vi "计算合并值32位.vi"(1 "数值LL":u8, 2 "数值L":u8, 3 "数值H":u8, 4 "数值HH":u8) -> (0 "合并数值":i32)   [LabVIEW 2016]
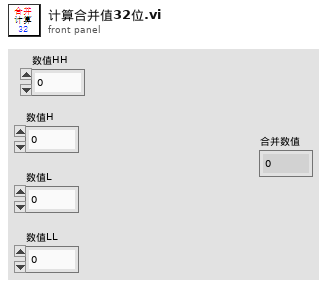
[diagram p1: front panel]
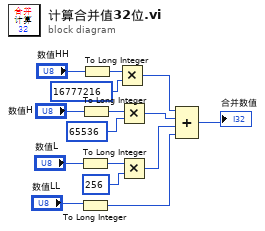
[diagram p0: block diagram]
diagram:
  n1 = To Long Integer(number="数值L") -> (32bit integer=w7:i32)
  n2 = To Long Integer(number="数值LL") -> (32bit integer=w2:i32)
  n3 = To Long Integer(number="数值H") -> (32bit integer=w13:i32)
  n4 = To Long Integer(number="数值HH") -> (32bit integer=w9:i32)
  n5 = Multiply(x=w9, y=16777216) -> (x*y=w5:i32)
  n6 = Multiply(x=w13, y=65536) -> (x*y=w4:i32)
  n7 = Multiply(x=w7, y=256) -> (x*y=w3:i32)
  n8 = Compound Arithmetic op=ADD(w5, w4, w3, w2) -> (→"合并数值":i32)
